vi "MineOrDumpBlocking.vi"(0 "Action":enum16{"Dump", "Mine"}(ring)) -> ()   [LabVIEW 2015, in "Overlord2017.lvlib"]
doc: "Mines or digs, as specified, by operating Mining and Dumping_r3.vi (or equivalent) by changing and watching global variables. Blocks execution until mining is completed."
uses:
  Overlord2017.lvlib
panel:
  out "Bucket State":string
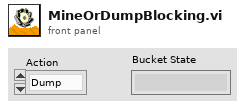
[diagram p1: front panel]
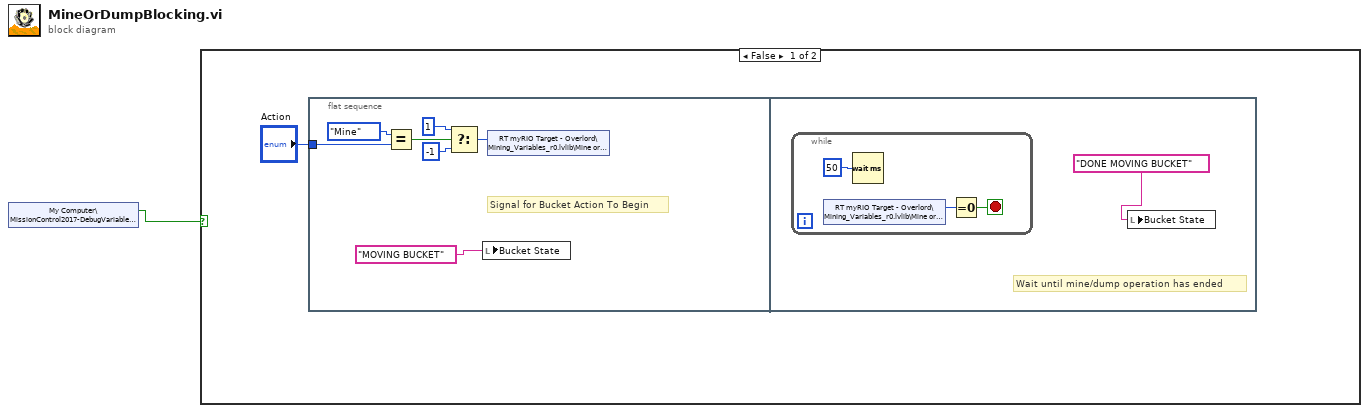
[diagram p0: block diagram]
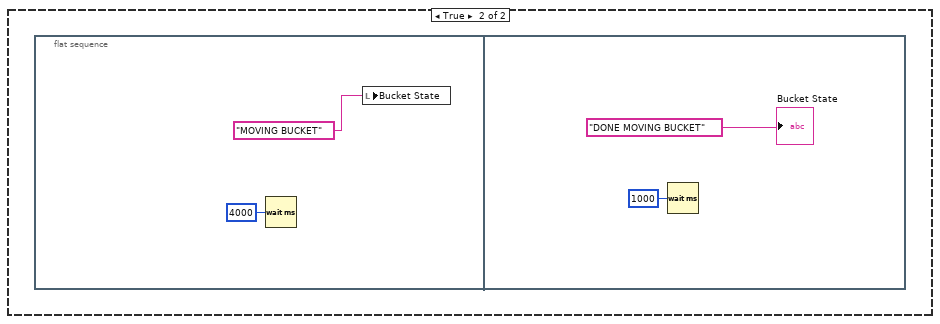
[diagram p2: hidden frame]
diagram:
  n1 = shared-variable "My Computer\\MissionControl2017-DebugVariables.lvlib\\DEBUG_BUCKET"() -> (w1:bool)  [unwired: 1 in, 1 out]
  n2 = case shown="False" w1 {
    frame False {
      n3 = flat-sequence {
        tunnel: "Action" -> [w5]
        frame #0 {
          # "Signal for Bucket Action To Begin"
          n4 = Equal?(x=enum16{"Dump", "Mine"}."Mine", y=w5) -> (x = y?=w6:bool)
          n5 = Select(t=1, s=w6, f=-1) -> (s? t:f=w9:i32)
          n6 = local write "Bucket State"("MOVING BUCKET") -> ()
          n7 = shared-variable "RT myRIO Target - Overlord\\Mining_Variables_r0.lvlib\\Mine or Dump"(w9) -> ()  [unwired: 1 in, 1 out]
        }
        frame #1 {
          # "Wait until mine/dump operation has ended"
          n8 = while {
            stop <- w13 stop-if-true
            n9 = shared-variable "RT myRIO Target - Overlord\\Mining_Variables_r0.lvlib\\Mine or Dump"() -> (w12:i16)  [unwired: 1 in, 1 out]
            n10 = Wait (ms)(milliseconds to wait=u32 50) -> ()  [unwired: 1 out]
            n11 = Equal To 0?(x=w12) -> (x = 0?=w13:bool)
          }
          n12 = local write "Bucket State"("DONE MOVING BUCKET") -> ()
        }
      }
    }
    frame True {
      n13 = flat-sequence {
        frame #0 {
          n14 = Wait (ms)(milliseconds to wait=u32 4000) -> ()  [unwired: 1 out]
          n15 = local write "Bucket State"("MOVING BUCKET") -> ()
        }
        frame #1 {
          n16 = Wait (ms)(milliseconds to wait=u32 1000) -> ()  [unwired: 1 out]
          "Bucket State" <- "DONE MOVING BUCKET"
        }
      }
    }
  }
